vi "WSTRING Byte Stream to String.vi"(8 "error in (no error)":errorcluster, 10 "Byte Stream":u8[](array[numeric])) -> (0 "error out":errorcluster, 2 "Value":string)   [LabVIEW 2018, in "TwinCAT ADS.lvclass"]
uses:
  TwinCAT ADS.lvclass
  TwinCAT.Ads
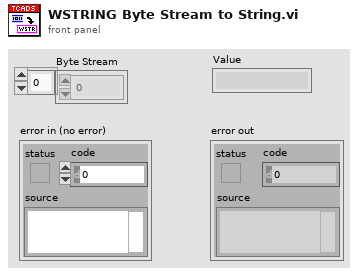
[diagram p1: front panel]
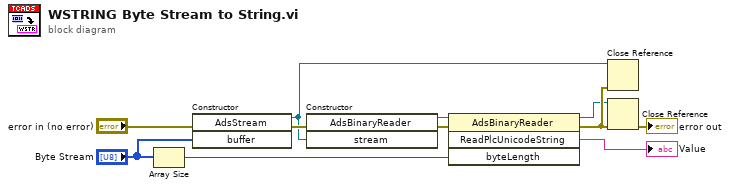
[diagram p0: block diagram]
diagram:
  n1 = Array Size(array="Byte Stream") -> (size(s)=w5:i32)
  n2 = constructor class="AdsStream"(error in="error in (no error)", "buffer"="Byte Stream") -> (reference out=w6:refnum<k24>, error out=w11:errorcluster)  [unwired: 2 in, 2 out]
  n3 = constructor class="AdsBinaryReader"(error in=w11, "stream"=w6) -> (reference out=w9:refnum<k24>, error out=w10:errorcluster)  [unwired: 2 in, 2 out]
  n4 = invoke class="AdsBinaryReader" method="ReadPlcUnicodeString"(reference=w9, error in=w10, "byteLength"=w5) -> (reference out=w7:refnum<k24>, error out=w8:errorcluster, "ReadPlcUnicodeString"=→"Value":string)  [unwired: 1 in, 1 out]
  n5 = Close Reference(reference=w6, error in (no error)=w8) -> ()  [unwired: 1 out]
  n6 = Close Reference(reference=w7, error in (no error)=w8) -> (error out=→"error out":errorcluster)
